vi "emi_Simple Variant Info.vi"(1 "use system decimal point (T)":bool=TRUE, 7 "Anything":variant, 9 "precision (12)":i16=12, 11 "error in(no error)":errorcluster, 12 "Exponential (T)":bool=TRUE) -> (4 "Name":string, 8 "String Value":string, 10 "Type":T1, 15 "error out":errorcluster)   [LabVIEW 2011]
doc: "Returns a textual representation of a data value, and the name, and data type of the data.\n\nUse system decimal point defines the decimal separator for floating point dat types. If TRUE (default), the decimal separator uses the localized decimal separator. If FALSE, the decimal separator is a period. \n \nPrecision The function rounds the number of digits after the decimal point of the output string to precision. If precision is 0, the output string does not contain a decimal point and contains at most three digits of the mantissa. The default is 12.\n\nExponential(T). If true, use exponential reprecentation of floating point values.\n\nSupports al data types except:\nVariant\nPicture\nTag\nArray\nWaveform\nDigital Waveform\nDigital Data\nExpressData\nRefnum\nExternal Data\nVI\nPoly VI\nLabview Class Instance\nFixed point\nCluster\n\nThis is intended for use with ini files, but may be adapted to other uses.\n\nOn error: Takes no action"
uses:
  <vilib>/Utility/VariantDataType/Type.ctl
  Error/emi_Create Error.vi
  <vilib>/Utility/VariantDataType/VariantType.lvlib
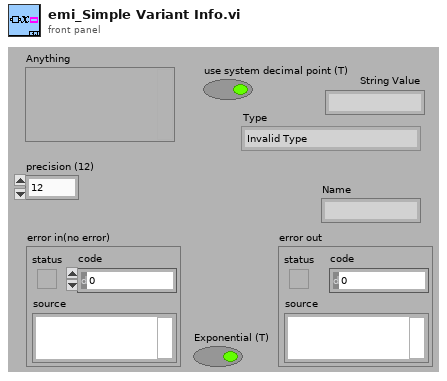
[diagram p1: front panel]
types:
  T1 = typedef "VariantType.lvlib/Type.ctl" = enum8{"Invalid Type", "Void", "I8", "I16", "I32", "I64", "U8", "U16", "U32", "U64", "Single Float", "Double Float", "Extended Float", "Single Complex", "Double Complex", "Extended Complex", "Enum U8", "Enum U16", "Enum U32", "Enum U64", "Single Float With Unit", "Double Float With Unit", "Extended Float With Unit", "Single Complex with Unit", "Double Complex with Unit", "Extended Complex with Unit", "Boolean", "String", "Path", "Picture", "Tag", "Array", "Cluster", "Variant", "LV Variant", "Waveform", "Timestamp", "Digital Waveform", "Digital Data", "ExpressData", "Refnum", "External Data", "VI", "Poly VI", "LabVIEW Class Instance", "Fixed Point"}
  T2 = typedef "VariantType.lvlib/UnitInfo.ctl" = cluster{"UnitType":T3, "Exponent":i16}
  T3 = typedef "VariantType.lvlib/UnitType.ctl" = enum16{"Radians", "Steradians", "Seconds", "Meters", "Kilograms", "Amperes", "Kelvins", "Moles", "Candelas", "InvalidUnit"}
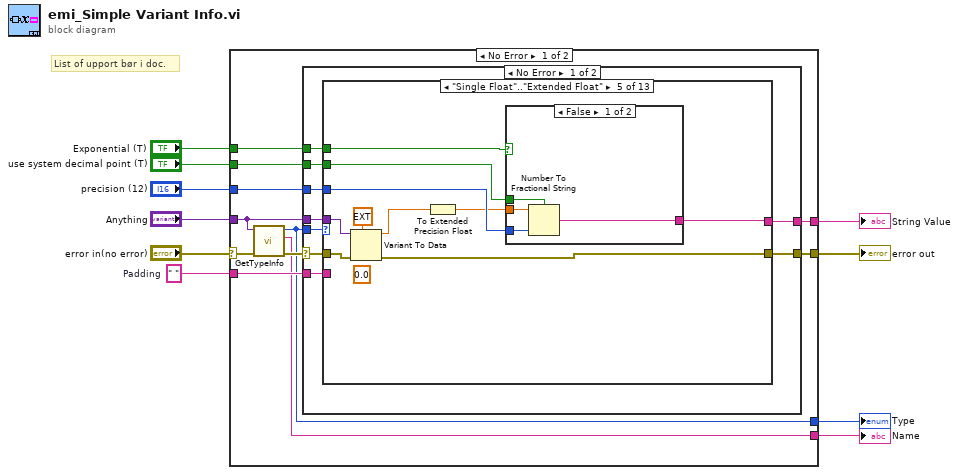
[diagram p0: block diagram]
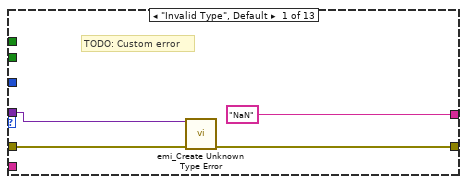
[diagram p2: hidden frame]
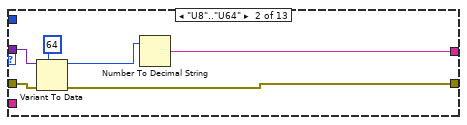
[diagram p3: hidden frame]
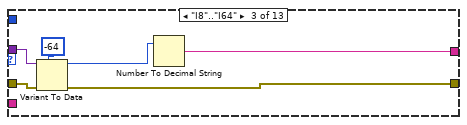
[diagram p4: hidden frame]
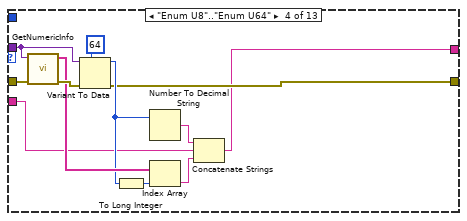
[diagram p5: hidden frame]
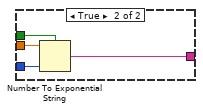
[diagram p6: hidden frame]
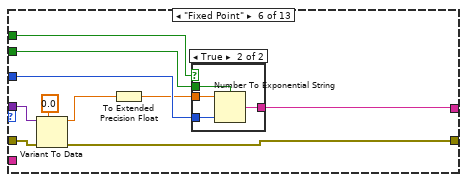
[diagram p7: hidden frame]
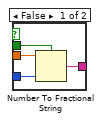
[diagram p8: hidden frame]
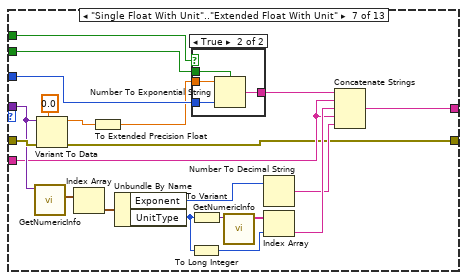
[diagram p9: hidden frame]
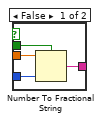
[diagram p10: hidden frame]
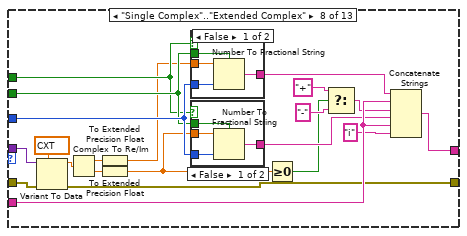
[diagram p11: hidden frame]
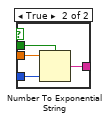
[diagram p12: hidden frame]
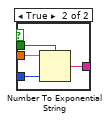
[diagram p13: hidden frame]
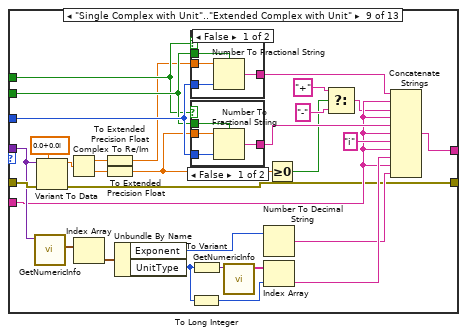
[diagram p14: hidden frame]
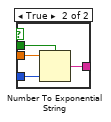
[diagram p15: hidden frame]
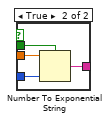
[diagram p16: hidden frame]
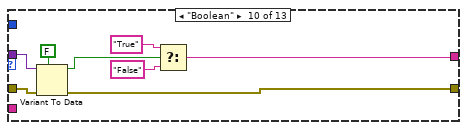
[diagram p17: hidden frame]
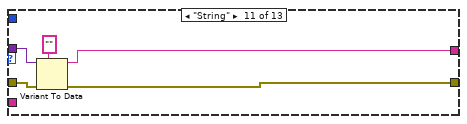
[diagram p18: hidden frame]
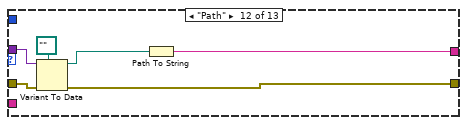
[diagram p19: hidden frame]
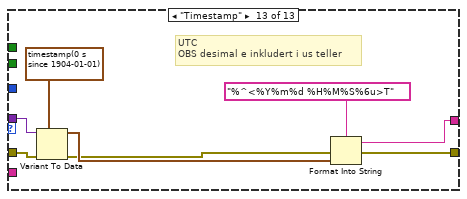
[diagram p20: hidden frame]
diagram:
  w9 = " "  # Padding
  # "List of upport bør i doc."
  n1 = case shown="No Error" "error in(no error)" {
    selector: "error in(no error)" -> [w14 w238]
    tunnel: [w21 w238] -> w10
    tunnel: w9 -> [w20 _]
    tunnel: [w19 ""] -> w8
    tunnel: "Exponential (T)" -> [w18 _]
    tunnel: "use system decimal point (T)" -> [w17 _]
    tunnel: "precision (12)" -> [w16 _]
    tunnel: "Anything" -> [w15 _]
    tunnel: [w12 "" ("Name")] -> w1
    tunnel: [w11 Type."Invalid Type" ("Type Enum")] -> w2
    frame No Error {
      n2 = call <vilib>:"GetTypeInfo.vi"("error in (no error)"=w14, "Variant"=w15) -> ("error out"=w13:errorcluster, "Name"=w12:string, "Type Enum"=w11:T1)  [unwired: 5 in, 2 out]
      n3 = case shown="No Error" w13 {
        selector: w13 -> [w22 w235]
        tunnel: [w30 w235] -> w21
        tunnel: w20 -> [w29 _]
        tunnel: [w28 ""] -> w19
        tunnel: w18 -> [w27 _]
        tunnel: w17 -> [w26 _]
        tunnel: w16 -> [w25 _]
        tunnel: w11 -> [w24 _]
        tunnel: w15 -> [w23 _]
        frame No Error {
          n4 = case shown="\"Single Float\"..\"Extended Float\"" w24 {
            tunnel: w23 -> [w32 w38 w44 w55 w66 w84 w107 w142 w182 w213 w218 w224 w232]
            tunnel: w22 -> [w33 w39 w45 w57 w67 w85 w114 w143 w189 w214 w219 w225 w233]
            tunnel: [w31 w37 w43 w48 w65 w83 w97 w136 w164 w211 w216 w222 w227] -> w30
            tunnel: w29 -> [_ _ _ w49 _ _ w103 w137 w168 _ _ _ _]
            tunnel: ["NaN" w35 w41 w47 w60 w78 w96 w135 w163 w207 w215 w220 w226] -> w28
            tunnel: w27 -> [_ _ _ _ w62 w80 w101 w138 w173 _ _ _ _]
            tunnel: w26 -> [_ _ _ _ w64 w82 w100 w139 w174 _ _ _ _]
            tunnel: w25 -> [_ _ _ _ w63 w81 w102 w140 w175 _ _ _ _]
            frame "Invalid Type", Default {
              # "TODO: Custom error"
              n5 = call "emi_Create Unknown Type Error.vi"("Anything"=w32, "error IO"=w33) -> ("error out"=w31:errorcluster)  [unwired: 13 in]
            }
            frame "U8".."U64" {
              n6 = Variant To Data(error in=w39, type=u64 64, Variant=w38) -> (data=w36:u64, error out=w37:errorcluster)
              n7 = Number To Decimal String(number=w36) -> (decimal integer string=w35:string)  [unwired: 1 in]
            }
            frame "I8".."I64" {
              n8 = Variant To Data(error in=w45, type=i64 -64, Variant=w44) -> (data=w42:i64, error out=w43:errorcluster)
              n9 = Number To Decimal String(number=w42) -> (decimal integer string=w41:string)  [unwired: 1 in]
            }
            frame "Enum U8".."Enum U64" {
              n10 = call <vilib>:"GetNumericInfo.vi"("error in (no error)"=w57, "Variant"=w55) -> ("error out"=w56:errorcluster, "EnumNames"=w54:string[])  [unwired: 6 in, 2 out]
              n11 = Variant To Data(error in=w56, type=u64 64, Variant=w55) -> (data=w51:u64, error out=w48:errorcluster)
              n12 = To Long Integer(number=w51) -> (32bit integer=w53:i32)
              n13 = Number To Decimal String(number=w51) -> (decimal integer string=w50:string)  [unwired: 1 in]
              n14 = Index Array(array=w54, index=w53) -> (element=w52:string)
              n15 = Concatenate Strings(w50, w49, w52) -> (w47:string)
            }
            frame "Single Float".."Extended Float" {
              (unwired) sgl 0.0
              n16 = Variant To Data(error in=w67, type=ext 0.0, Variant=w66) -> (data=w61:ext, error out=w65:errorcluster)
              n17 = To Extended Precision Float(1:w61) -> (0:w59:ext)
              n18 = case shown="False" w62 {
                tunnel: w64 -> [w71 w76]
                tunnel: w63 -> [w72 w75]
                tunnel: [w70 w74] -> w60
                tunnel: w59 -> [w69 w73]
                frame False {
                  n19 = Number To Fractional String(use system decimal point (T)=w71, number=w69, precision (6)=w72) -> (F-format string=w70:string)  [unwired: 1 in]
                }
                frame True {
                  n20 = Number To Exponential String(number=w73, precision (6)=w75, 1:w76) -> (E-format string=w74:string)  [unwired: 1 in]
                }
              }
            }
            frame "Fixed Point" {
              n21 = Variant To Data(error in=w85, type=sgl 0.0, Variant=w84) -> (data=w79:sgl, error out=w83:errorcluster)
              n22 = To Extended Precision Float(1:w79) -> (0:w77:ext)
              n23 = case shown="True" w80 {
                tunnel: w82 -> [w89 w94]
                tunnel: w81 -> [w90 w93]
                tunnel: [w88 w92] -> w78
                tunnel: w77 -> [w87 w91]
                frame False {
                  n24 = Number To Fractional String(use system decimal point (T)=w89, number=w87, precision (6)=w90) -> (F-format string=w88:string)  [unwired: 1 in]
                }
                frame True {
                  n25 = Number To Exponential String(number=w91, precision (6)=w93, 1:w94) -> (E-format string=w92:string)  [unwired: 1 in]
                }
              }
            }
            frame "Single Float With Unit".."Extended Float With Unit" {
              n26 = call <vilib>:"GetNumericInfo.vi"("Variant"=w107) -> ("Units"=w108:T2[])  [unwired: 7 in, 3 out]
              n27 = Variant To Data(error in=w114, type=sgl 0.0, Variant=w107) -> (data=w99:sgl, error out=w97:errorcluster)
              n28 = Index Array(array=w108) -> (element=w109:T2)  [unwired: 1 in]
              n29 = To Extended Precision Float(1:w99) -> (0:w95:ext)
              n30 = Unbundle By Name(w109) -> ("Exponent"=w106:i16, "UnitType"=w112:T3)
              n31 = To Long Integer(number=w112) -> (32bit integer=w113:i32)
              n32 = case shown="True" w101 {
                tunnel: w100 -> [w118 w123]
                tunnel: w102 -> [w119 w122]
                tunnel: [w117 w121] -> w98
                tunnel: w95 -> [w116 w120]
                frame False {
                  n33 = Number To Fractional String(use system decimal point (T)=w118, number=w116, precision (6)=w119) -> (F-format string=w117:string)  [unwired: 1 in]
                }
                frame True {
                  n34 = Number To Exponential String(number=w120, precision (6)=w122, 1:w123) -> (E-format string=w121:string)  [unwired: 1 in]
                }
              }
              n35 = To Variant(anything=w112) -> (Variant=w110:variant)
              n36 = call <vilib>:"GetNumericInfo.vi"("Variant"=w110) -> ("EnumNames"=w111:string[])  [unwired: 7 in, 3 out]
              n37 = Number To Decimal String(number=w106) -> (decimal integer string=w104:string)  [unwired: 1 in]
              n38 = Index Array(array=w111, index=w113) -> (element=w105:string)
              n39 = Concatenate Strings(w98, w103, w105, w103, w104) -> (w96:string)
            }
            frame "Single Complex".."Extended Complex" {
              n40 = Variant To Data(error in=w143, type=cxt 0.0+0.0i, Variant=w142) -> (data=w141:cxt, error out=w136:errorcluster)
              n41 = Complex To Re/Im(x + iy=w141) -> (x=w133:ext, y=w128:ext)
              n42 = To Extended Precision Float(1:w133) -> (0:w125:ext)
              n43 = To Extended Precision Float(1:w128) -> (0:w124:ext)
              n44 = case shown="False" w138 {
                tunnel: w139 -> [w155 w160]
                tunnel: w140 -> [w156 w159]
                tunnel: [w154 w158] -> w132
                tunnel: w125 -> [w153 w157]
                frame False {
                  n45 = Number To Fractional String(use system decimal point (T)=w155, number=w153, precision (6)=w156) -> (F-format string=w154:string)  [unwired: 1 in]
                }
                frame True {
                  n46 = Number To Exponential String(number=w157, precision (6)=w159, 1:w160) -> (E-format string=w158:string)  [unwired: 1 in]
                }
              }
              n47 = case shown="False" w138 {
                tunnel: w139 -> [w147 w152]
                tunnel: w140 -> [w148 w151]
                tunnel: [w146 w150] -> w129
                tunnel: w124 -> [w145 w149]
                frame False {
                  n48 = Number To Fractional String(use system decimal point (T)=w147, number=w145, precision (6)=w148) -> (F-format string=w146:string)  [unwired: 1 in]
                }
                frame True {
                  n49 = Number To Exponential String(number=w149, precision (6)=w151, 1:w152) -> (E-format string=w150:string)  [unwired: 1 in]
                }
              }
              n50 = Greater Or Equal To 0?(x=w124) -> (x >= 0?=w127:bool)
              n51 = Select(t="+" ("string"), s=w127, f="-" ("string")) -> (s? t:f=w126:string)
              n52 = Concatenate Strings(w132, w137, w126, w129, w137, "i" ("string")) -> (w135:string)
            }
            frame "Single Complex with Unit".."Extended Complex with Unit" {
              n53 = call <vilib>:"GetNumericInfo.vi"("Variant"=w182) -> ("Units"=w183:T2[])  [unwired: 7 in, 3 out]
              n54 = Variant To Data(error in=w189, type=csg 0.0+0.0i, Variant=w182) -> (data=w178:csg, error out=w164:errorcluster)
              n55 = Complex To Re/Im(x + iy=w178) -> (x=w176:sgl, y=w167:sgl)
              n56 = Index Array(array=w183) -> (element=w184:T2)  [unwired: 1 in]
              n57 = To Extended Precision Float(1:w176) -> (0:w162:ext)
              n58 = To Extended Precision Float(1:w167) -> (0:w161:ext)
              n59 = Unbundle By Name(w184) -> ("Exponent"=w181:i16, "UnitType"=w187:T3)
              n60 = case shown="False" w173 {
                tunnel: w174 -> [w201 w206]
                tunnel: w175 -> [w202 w205]
                tunnel: [w200 w204] -> w172
                tunnel: w162 -> [w199 w203]
                frame False {
                  n61 = Number To Fractional String(use system decimal point (T)=w201, number=w199, precision (6)=w202) -> (F-format string=w200:string)  [unwired: 1 in]
                }
                frame True {
                  n62 = Number To Exponential String(number=w203, precision (6)=w205, 1:w206) -> (E-format string=w204:string)  [unwired: 1 in]
                }
              }
              n63 = case shown="False" w173 {
                tunnel: w174 -> [w193 w198]
                tunnel: w175 -> [w194 w197]
                tunnel: [w192 w196] -> w169
                tunnel: w161 -> [w191 w195]
                frame False {
                  n64 = Number To Fractional String(use system decimal point (T)=w193, number=w191, precision (6)=w194) -> (F-format string=w192:string)  [unwired: 1 in]
                }
                frame True {
                  n65 = Number To Exponential String(number=w195, precision (6)=w197, 1:w198) -> (E-format string=w196:string)  [unwired: 1 in]
                }
              }
              n66 = To Long Integer(number=w187) -> (32bit integer=w188:i32)
              n67 = To Variant(anything=w187) -> (Variant=w185:variant)
              n68 = call <vilib>:"GetNumericInfo.vi"("Variant"=w185) -> ("EnumNames"=w186:string[])  [unwired: 7 in, 3 out]
              n69 = Number To Decimal String(number=w181) -> (decimal integer string=w179:string)  [unwired: 1 in]
              n70 = Index Array(array=w186, index=w188) -> (element=w180:string)
              n71 = Greater Or Equal To 0?(x=w161) -> (x >= 0?=w166:bool)
              n72 = Select(t="+" ("string"), s=w166, f="-" ("string")) -> (s? t:f=w165:string)
              n73 = Concatenate Strings(w172, w168, w165, w168, w169, w168, "i" ("string"), w168, w180, w168, w179) -> (w163:string)
            }
            frame "Boolean" {
              n74 = Variant To Data(error in=w214, type=FALSE, Variant=w213) -> (data=w210:bool, error out=w211:errorcluster)
              n75 = Select(t="True", s=w210, f="False") -> (s? t:f=w207:string)
            }
            frame "String" {
              n76 = Variant To Data(error in=w219, type="", Variant=w218) -> (data=w215:string, error out=w216:errorcluster)
            }
            frame "Path" {
              n77 = Variant To Data(error in=w225, type=path "", Variant=w224) -> (data=w221:path, error out=w222:errorcluster)
              n78 = Path To String(path=w221) -> (string=w220:string)
            }
            frame "Timestamp" {
              # "UTC\nOBS desimal e inkludert i us teller"
              n79 = Variant To Data(error in=w233, type=timestamp(0 s since 1904-01-01), Variant=w232) -> (data=w229:timestamp, error out=w228:errorcluster)
              n80 = Format Into String(format string="%^<%Y%m%d %H%M%S%6u>T", error in=w228, w229) -> (resulting string=w226:string, error out=w227:errorcluster)  [unwired: 1 in]
            }
          }
        }
        frame Error {
        }
      }
    }
    frame Error {
    }
  }
  "error out" <- w10
  "String Value" <- w8
  "Type" <- w2
  "Name" <- w1
